vi "Accumulated Sector Intensity.vi"() -> ()   [LabVIEW 2013]
panel:
  in  "Total Wing Sectors":u8 max=32
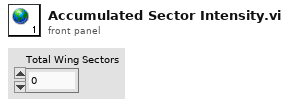
[diagram p1: front panel]
diagram:
